vi "SVL Limit Testing (peaks) (scalar limits).vi"(8 "error in (no error)":errorcluster, 9 "lower limit":dbl=-inf format="%.2f", 10 "upper limit":dbl=inf format="%.2f", 11 "peaks in":cluster{"freq. or order":dbl, "amplitude":dbl}[](array[cluster]) {"amplitude" format="%.2f"; "freq. or order" format="%.2f"}) -> (0 "error out":errorcluster, 1 "output values":cluster{"frequencies":dbl[], "spectrum":dbl[]}[](graph), 2 "test results":bool[](array[boolean]), 3 "test passed?":bool)   [LabVIEW 2017, in "SoundVib_LimitTest.lvlib"]
doc: "Performs limit testing on waveforms, spectra, XY data, identified peaks, or scalar measurements. You can specify an upper and lower boundary of the envelope to define a pass range. This VI uses the defined pass range to test the input signal. VI outputs apply only to the current input signal. You can wire output values to a graph to view the limits, signal, and failures. Wire data to the<B> signal in</B> input to determine the polymorphic instance to use or manually select the instance."
uses:
  <vilib>/addons/Sound and Vibration/svt_Limit Test/SoundVib_LimitTest.lvlib
  <vilib>/addons/_NISVFA/_Shared subVIs/Common/svc_Convert Array of Peaks to X and Y Arrays.vi
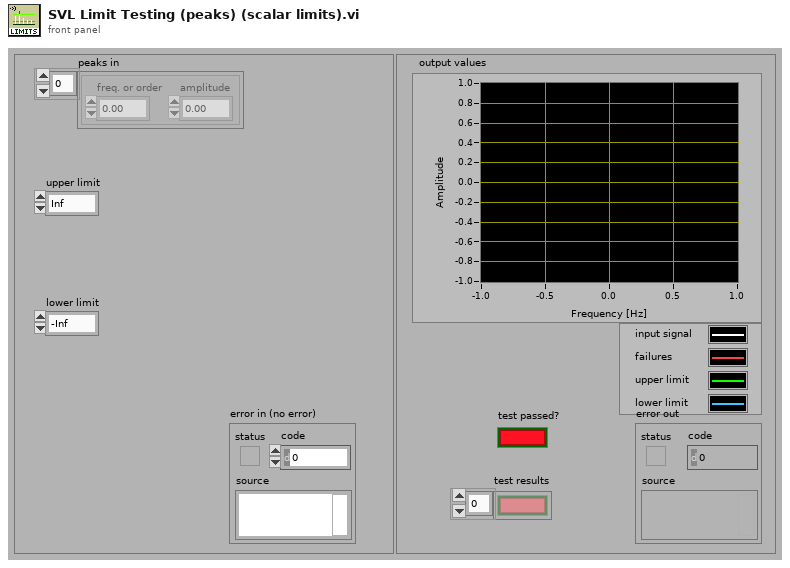
[diagram p1: front panel]
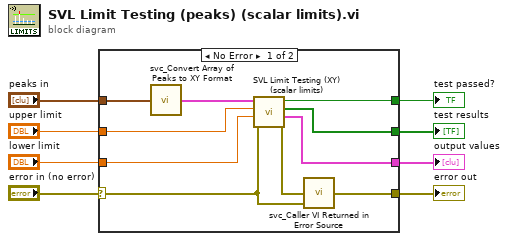
[diagram p0: block diagram]
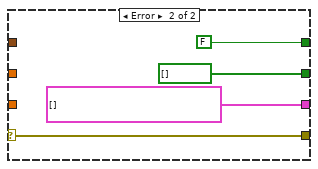
[diagram p2: hidden frame]
diagram:
  n1 = case shown="No Error" "error in (no error)" {
    selector: "error in (no error)" -> [w9 w22]
    tunnel: [w18 w22] -> w7
    tunnel: "peaks in" -> [w15 _]
    tunnel: "upper limit" -> [w14 _]
    tunnel: "lower limit" -> [w13 _]
    tunnel: [w12 FALSE ("test passed?")] -> w3
    tunnel: [w11 bool[] [] ("test results")] -> w2
    tunnel: [w10 cluster{"X":dbl[], "Y":dbl[]}[] [] ("output values")] -> w1
    frame No Error {
      n2 = call <vilib>:"svc_Convert Array of Peaks to XY Format.vi"("peaks"=w15) -> ("peaks"=w17:cluster{"X":dbl[], "Y":dbl[]})  [unwired: 4 in]
      n3 = call <vilib>:"SVL Limit Testing (XY) (scalar limits).vi"("error in (no error)"=w9, "lower limit"=w13, "upper limit"=w14, "signal in"=w17) -> ("error out"=w16:errorcluster, "output values"=w10:cluster{"frequencies":dbl[], "spectrum":dbl[]}[], "test results"=w11:bool[], "test passed?"=w12:bool)  [unwired: 4 in]
      n4 = call <vilib>:"svc_Caller VI Returned in Error Source.vi"("warning input to caller"=w9, "error in (no error)"=w16) -> ("error out"=w18:errorcluster)  [unwired: 3 in]
    }
    frame Error {
    }
  }
  "error out" <- w7
  "output values" <- w1
  "test passed?" <- w3
  "test results" <- w2
